vi "Timer Tick Set Time.vi"(5 "Seconds till stop (ms)":dbl, 6 "Seconds till stop (S)":dbl) -> (1 "current time":timestamp, 2 "Finish Time":timestamp)   [LabVIEW 2023]
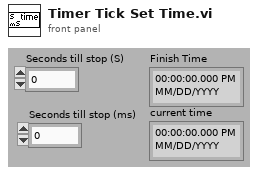
[diagram p1: front panel]
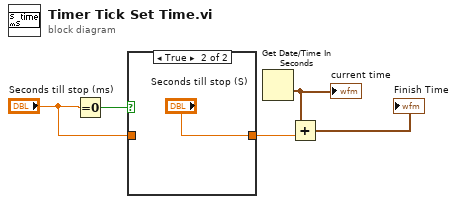
[diagram p0: block diagram]
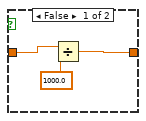
[diagram p2: hidden frame]
diagram:
  n1 = Equal To 0?(x="Seconds till stop (ms)") -> (x = 0?=w4:bool)
  n2 = case shown="True" w4 {
    tunnel: [w8 "Seconds till stop (S)"] -> w5
    tunnel: "Seconds till stop (ms)" -> [w7 _]
    frame False {
      n3 = Divide(x=w7, y=1000.0) -> (x/y=w8:dbl)
    }
    frame True {
    }
  }
  n4 = Get Date/Time In Seconds() -> (seconds since 1Jan1904=w2:timestamp)
  "current time" <- w2
  n5 = Add(x=w2, y=w5) -> (x+y=→"Finish Time":timestamp)
